vi "FTW-TestExecutive-Sequence-Serialize.vi"(0 "Sequence":T1[](array[typedef]) {"Results"."Start Time" format="%<%Y-%m-%d %H:%M:%S%03u>T"; "Results"."Elapsed Time" format="%<%H:%M:%S%3u>t"; "Elapsed Time" format="%<%H:%M:%S%3u>t"}, 11 "error in":errorcluster) -> (4 "JSON":string, 15 "error out":errorcluster)   [LabVIEW 2015]
doc: "Can be used to interpret the following messages\n\nSequenceLoaded\nSequenceComplete\nStepChange"
uses:
  FTW-TestExecutive-Step.ctl
  FTW-TestExecutive-Step-State.ctl
  FTW-TestExecutive-Results.ctl
  source/JSON/FTW-JSON-JoinMode.ctl
  source/container/FTW-Container.lvclass
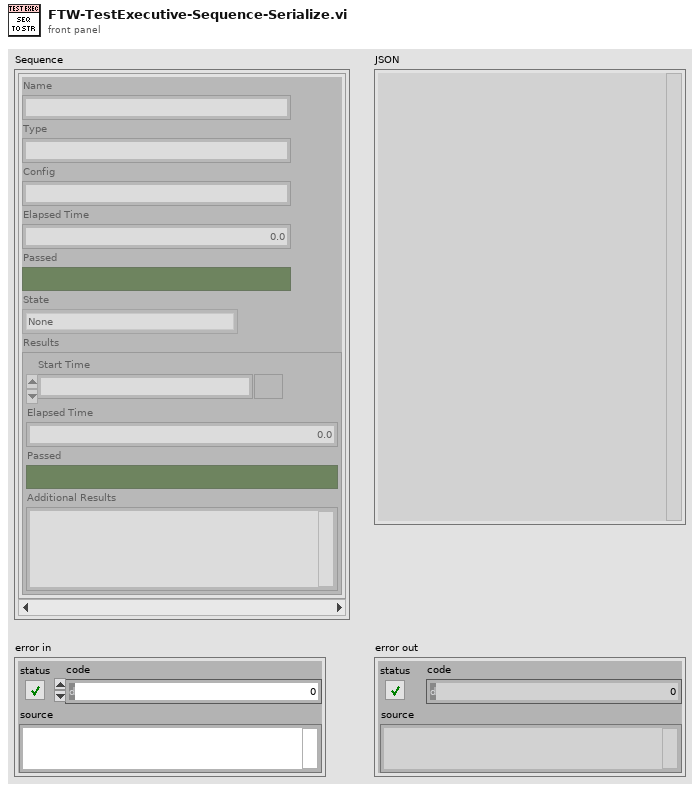
[diagram p1: front panel]
types:
  T1 = typedef "FTW-TestExecutive-Step.ctl" = cluster{"Name":string, "Type":string, "Config":string, "Elapsed Time":dbl, "Passed":bool, "State":T2, "Results":T3}
  T2 = typedef "FTW-TestExecutive-Step-State.ctl" = enum8{"None", "Failed", "Passed", "Timed out", "Aborted"}
  T3 = typedef "FTW-TestExecutive-Results.ctl" = cluster{"Start Time":timestamp, "Elapsed Time":dbl, "Passed":bool, "Additional Results":string}
  T4 = typedef "FTW-JSON-JoinMode.ctl" = enum32{"Upsert", "Update Only", "Insert Only"}
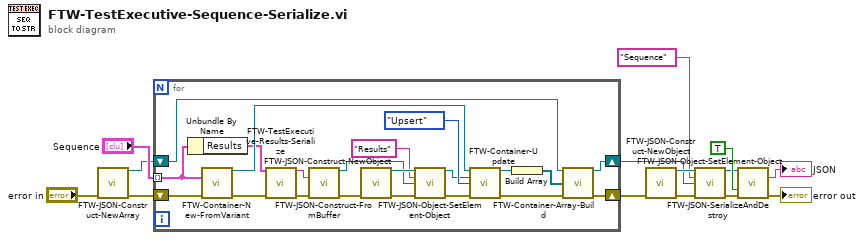
[diagram p0: block diagram]
diagram:
  n1 = call "FTW-JSON-Construct-NewArray.vi"("error in"="error in") -> ("JSON"=w10:refnum<class "FTW-Container.lvclass">, "error out"=w11:errorcluster)  [unwired: 13 in]
  n2 = for {
    tunnel: "Sequence" -> [w33] mode=indexing
    shift-right: [w24] -> w12
    shift-left: w11 -> [w25]
    shift-right: [w21] -> w6
    shift-left: w10 -> [w22]
    n3 = Unbundle By Name(w33) -> ("Results"=w31:T3)
    n4 = call "FTW-Container-New-FromVariant.vi"("Variant"=w33, "error in"=w25) -> ("FTW-Container"=w35:refnum<class "FTW-Container.lvclass">, "error out"=w29:errorcluster)  [unwired: 12 in]
    n5 = call "FTW-TestExecutive-Results-Serialize.vi"("Results"=w31, "error in (no error)"=w29) -> ("Serialized Results"=w32:string, "error out"=w30:errorcluster)  [unwired: 12 in]
    n6 = call "FTW-JSON-Construct-FromBuffer.vi"("JSON String (UTF-8)"=w32, "error in"=w30) -> ("JSON"=w16:refnum<class "FTW-Container.lvclass">, "error out"=w28:errorcluster)  [unwired: 12 in]
    n7 = call "FTW-JSON-Construct-NewObject.vi"("error in"=w28) -> ("JSON"=w18:refnum<class "FTW-Container.lvclass">, "error out"=w20:errorcluster)  [unwired: 13 in]
    n8 = call "FTW-JSON-Object-SetElement-Object.vi"("JSON Object"=w18, "Key"="Results", "JSON Sub-Object"=w16, "error in"=w20) -> ("JSON Root Object"=w17:refnum<class "FTW-Container.lvclass">, "error out"=w19:errorcluster)  [unwired: 10 in]
    n9 = call "FTW-Container-Update.vi"("FTW-Container In"=w35, "Other Container"=w17, "Join Mode"=FTW-JSON-JoinMode."Upsert", "error in"=w19) -> ("Updated Container"=w27:refnum<class "FTW-Container.lvclass">, "error out"=w23:errorcluster)  [unwired: 10 in]
    n10 = Build Array(w27) -> (w26:refnum<class "FTW-Container.lvclass">[])
    n11 = call "FTW-Container-Array-Build.vi"("FTW-Container In"=w22, "Array Elements"=w26, "error in"=w23) -> ("FTW-Container Out"=w21:refnum<class "FTW-Container.lvclass">, "error out"=w24:errorcluster)  [unwired: 11 in]
  }
  n12 = call "FTW-JSON-Construct-NewObject.vi"("error in"=w12) -> ("JSON"=w7:refnum<class "FTW-Container.lvclass">, "error out"=w9:errorcluster)  [unwired: 13 in]
  n13 = call "FTW-JSON-Object-SetElement-Object.vi"("JSON Object"=w7, "Key"="Sequence", "JSON Sub-Object"=w6, "error in"=w9) -> ("JSON Root Object"=w2:refnum<class "FTW-Container.lvclass">, "error out"=w8:errorcluster)  [unwired: 10 in]
  n14 = call "FTW-JSON-SerializeAndDestroy.vi"("JSON"=w2, "Pretty Print"=TRUE, "error in"=w8) -> ("JSON String (UTF-8)"=→"JSON":string, "error out"=→"error out":errorcluster)  [unwired: 11 in]
